vi "CloseTCP.vi"() -> ()   [LabVIEW 2020]
panel:
  in  "Error In":errorcluster
  out "error out":errorcluster
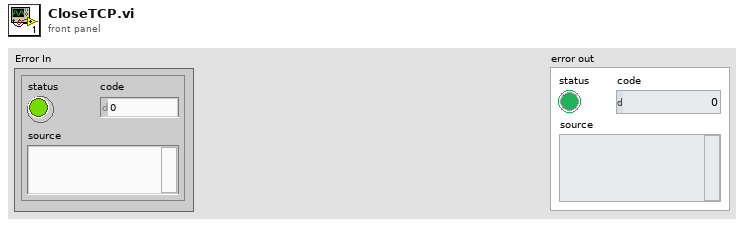
[diagram p1: front panel]
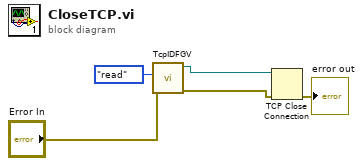
[diagram p0: block diagram]
diagram:
  n1 = call "TcpIDFGV.vi"("Error In"="Error In", "action"=enum16{"write", "read"}."read") -> ("Error Out"=w3:errorcluster, "connection ID out"=w4:refnum<k5>)  [unwired: 8 in]
  n2 = TCP Close Connection(connection ID=w4, error in (no error)=w3) -> (error out=→"error out":errorcluster)  [unwired: 1 in, 1 out]
